vi "S-Curve sub part.vi"(4 "1-(v_f/v)":dbl, 5 "v_i/v":dbl, 6 "1-(v_i/v)":dbl, 7 "x":dbl, 8 "4a/v":dbl, 9 "t-c2":dbl, 10 "c1":dbl, 11 "v":dbl) -> (3 "v_out":dbl)   [LabVIEW 2020]
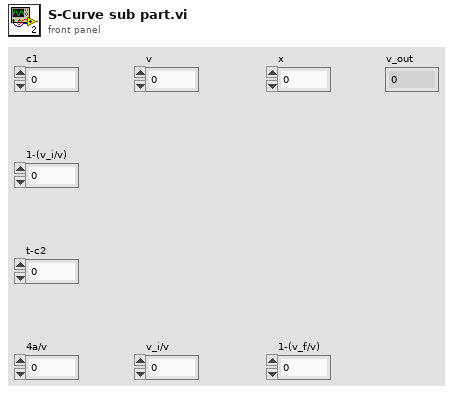
[diagram p1: front panel]
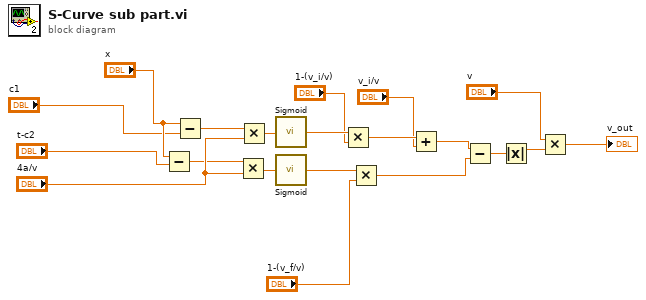
[diagram p0: block diagram]
diagram:
  n1 = Subtract(x="x", y="t-c2") -> (x-y=w7:dbl)
  n2 = Subtract(x="x", y="c1") -> (x-y=w6:dbl)
  n3 = Multiply(x=w7, y="4a/v") -> (x*y=w9:dbl)
  n4 = Multiply(x=w6, y="4a/v") -> (x*y=w8:dbl)
  n5 = call "Sigmoid.vi"("x"=w8) -> ("sigmoid(x)"=w16:dbl)
  n6 = call "Sigmoid.vi"("x"=w9) -> ("sigmoid(x)"=w17:dbl)
  n7 = Multiply(x=w16, y="1-(v_i/v)") -> (x*y=w19:dbl)
  n8 = Multiply(x=w17, y="1-(v_f/v)") -> (x*y=w18:dbl)
  n9 = Add(x=w19, y="v_i/v") -> (x+y=w20:dbl)
  n10 = Subtract(x=w20, y=w18) -> (x-y=w10:dbl)
  n11 = Absolute Value(x=w10) -> (abs(x)=w11:dbl)
  n12 = Multiply(x="v", y=w11) -> (x*y=→"v_out":dbl)
